vi "ConfigUtilities - Initialize Device Properties.vi"(8 "error in (no error)":errorcluster, 11 "Device Item Ref in":T1 format="%.0x") -> (0 "error out":errorcluster, 3 "Item Ref out":T1 format="%.0x")   [LabVIEW 2016, in "UDP-Custom-Device System Explorer.lvlib"]
doc: "Initialize the UDP Data Link custom device properties."
uses:
  UDP-Custom-Device System Explorer.lvlib
  <vilib>/NI Veristand/Custom Device API/Custom Device Item Ref.ctl
  Shared/Constants.vi
  <vilib>/NI Veristand/Custom Device API/Set Item Property (Boolean).vi
  <vilib>/NI Veristand/Custom Device API/Set Item Property (Path).vi
  <vilib>/NI VeriStand/Custom Device API/Custom Device API.lvlib
  Shared/UDP-Custom-Device Shared.lvlib
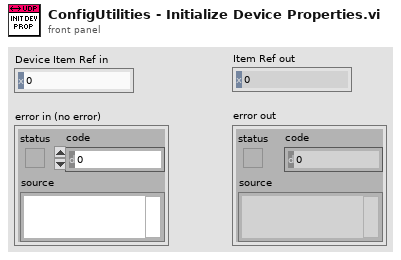
[diagram p1: front panel]
types:
  T1 = typedef "Custom Device API.lvlib/Custom Device Item Ref.ctl" = u64
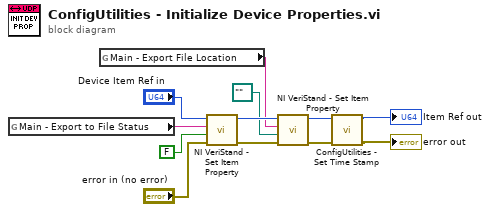
[diagram p0: block diagram]
diagram:
  n1 = global read "Constants.vi" "Main - Export to File Status"() -> (w5:string)
  n2 = global read "Constants.vi" "Main - Export File Location"() -> (w6:string)
  n3 = call-poly <vilib>:"NI VeriStand - Set Item Property.vi"("error in (no error)"="error in (no error)", "Value"=FALSE, "Property Name"=w5, "Item Ref in"="Device Item Ref in") -> ("error out"=w10:errorcluster, "Item Ref out"=w11:T1)  [unwired: 5 in, 1 out]
  n4 = call-poly <vilib>:"NI VeriStand - Set Item Property.vi"("error in (no error)"=w10, "Value"=path "", "Property Name"=w6, "Item Ref in"=w11) -> ("error out"=w1:errorcluster, "Item Ref out"=w2:T1)  [unwired: 5 in, 1 out]
  n5 = call "ConfigUtilities - Set Time Stamp.vi"("error in (no error)"=w1, "Device Item Ref in"=w2) -> ("error out"=→"error out":errorcluster, "Device Item Ref out"=→"Item Ref out":T1)  [unwired: 7 in, 1 out]
